vi "RP-VOA READ CALIBRATION.vi"(2 "error in (no error)":errorcluster, 3 "polynomial order":i32=2, 4 "file path":path) -> (0 "error out":errorcluster, 1 "Polynomial Coefficients":dbl[](array[numeric]))   [LabVIEW 2021]
uses:
  <vilib>/Utility/file.llb/Read Delimited Spreadsheet (DBL).vi
  <vilib>/Analysis/NI_AALPro.lvlib
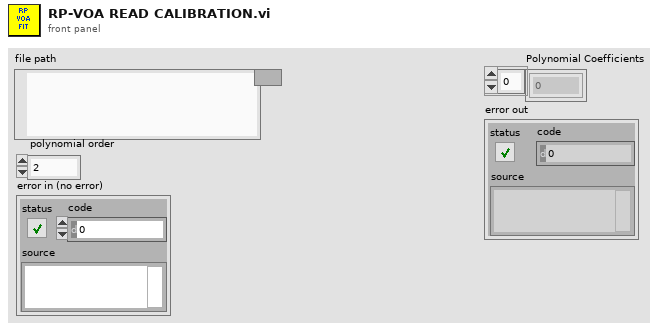
[diagram p1: front panel]
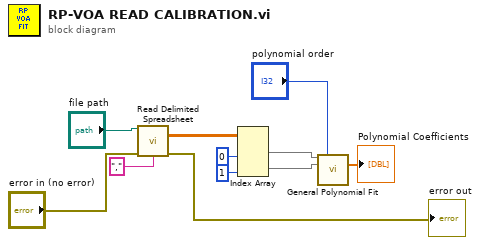
[diagram p0: block diagram]
diagram:
  n1 = call-poly <vilib>:"Read Delimited Spreadsheet.vi"("file path (dialog if empty)"="file path", "error in (no error)"="error in (no error)", "delimiter (\\t)"="," ("delimiter (\\t)")) -> ("all rows"=w9:dbl[][], "error out"=→"error out":errorcluster)  [unwired: 7 in, 4 out]
  n2 = Index Array(array=w9, index (col) #1=0 ("disabled index (col)"), index (col) #2=1 ("index (col)")) -> (element #1=w6:dbl[], element #2=w5:dbl[])  [unwired: 2 in]
  n3 = call <vilib>:"General Polynomial Fit.vi"("Y"=w6, "polynomial order"="polynomial order", "X"=w5) -> ("Polynomial Coefficients"=→"Polynomial Coefficients":dbl[])  [unwired: 9 in, 3 out]
